vi "Prompt for Password.vi"(11 "Pipe Path":path) -> ()   [LabVIEW 2020, in "NI_SSH.lvlib" / "OpenSSH Client.lvclass"]
uses:
  <vilib>/net/SSH/Client/OpenSSH/OpenSSH Client.lvclass
  <vilib>/Subprocess/Subprocess/Subprocess.lvclass
panel:
  in  "Cancel":bool
  in  "OK":bool
  in  "Password":string="\n\n\nmz3bq.ar" caption="Password:"
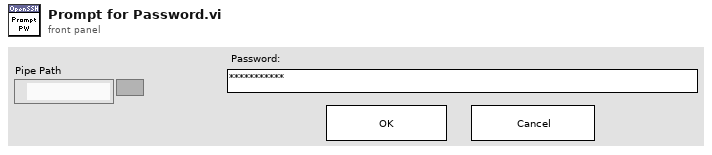
[diagram p1: front panel]
types:
  T1 = enum32{"Invalid", "Standard", "Closed", "Hidden", "Minimized", "Maximized"}
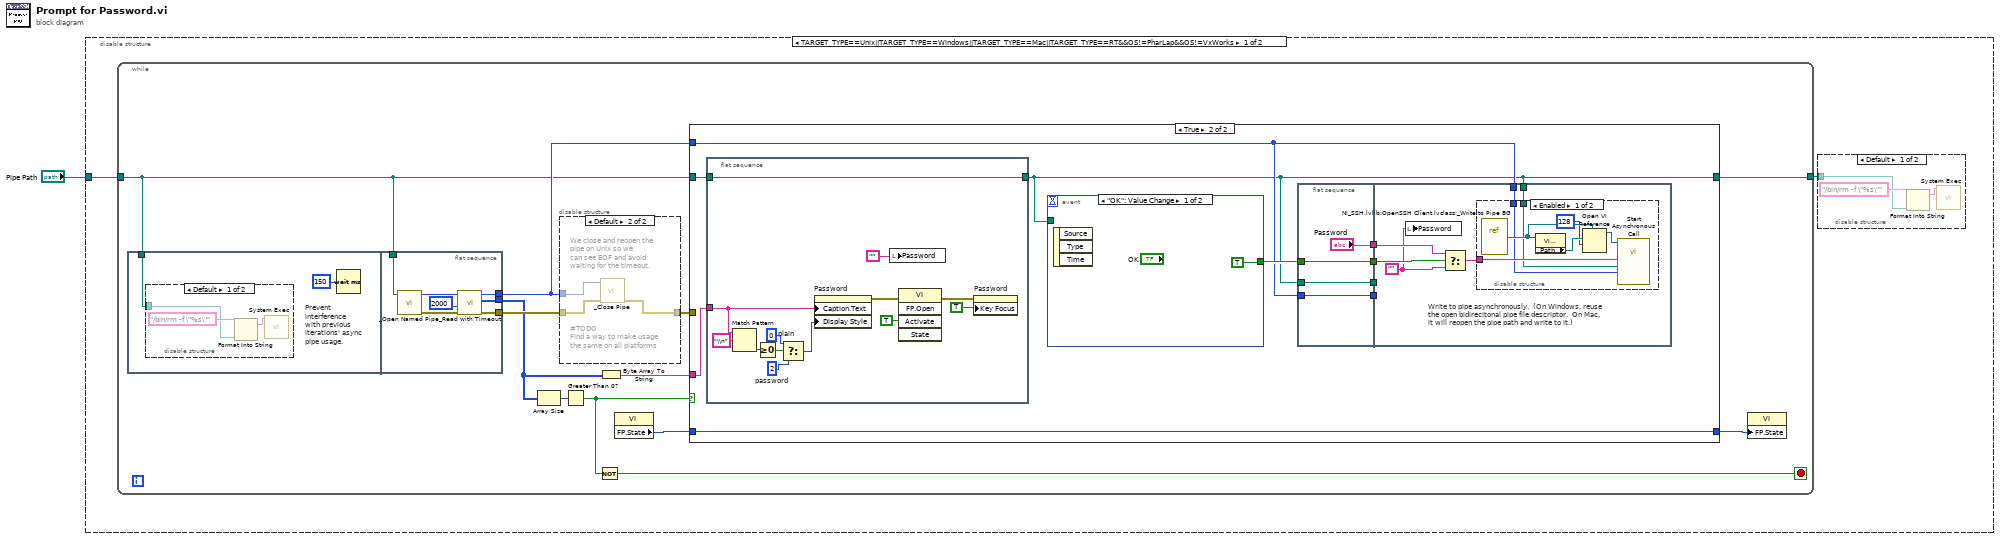
[diagram p0: block diagram]
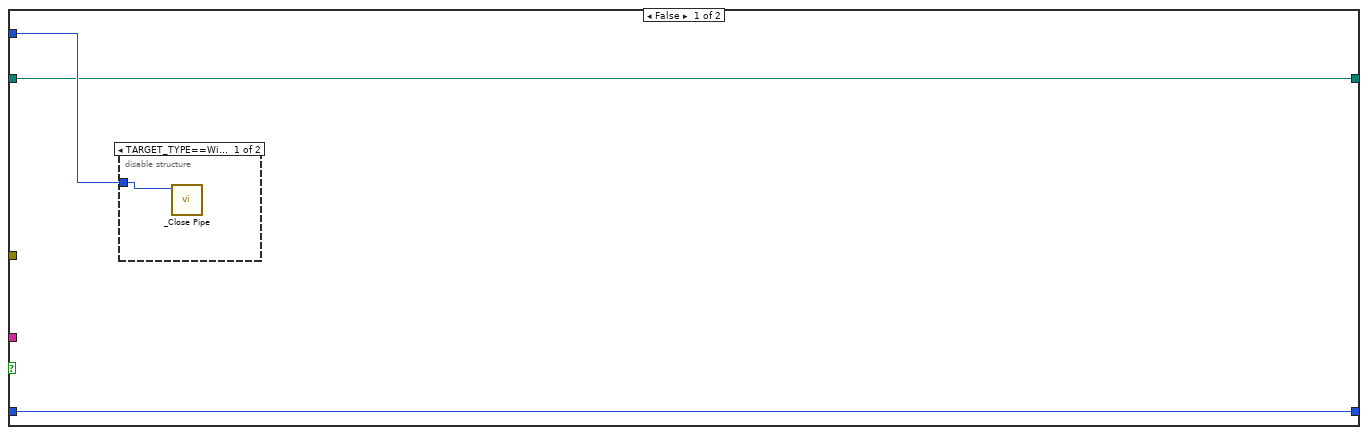
[diagram p5: hidden frame]
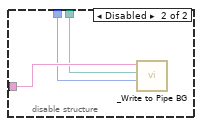
[diagram p7: hidden frame]
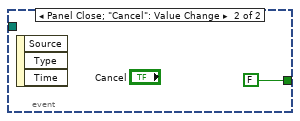
[diagram p8: hidden frame]
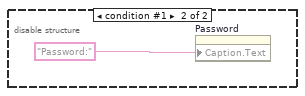
[diagram p9: hidden frame]
diagram:
  n1 = disable-structure "Conditional Disable Structure" shown="TARGET_TYPE==Unix||TARGET_TYPE==Windows||TARGET_TYPE==Mac||TARGET_TYPE==RT&&OS!=PharLap&&OS!=VxWorks" {
    disable-tunnel: "Pipe Path" -> [w3 _]
    frame condition #0 (active) {
      n2 = while {
        tunnel: w3 -> [w7]
        tunnel: [w8] -> w2
        stop <- w14 stop-if-true
        n3 = flat-sequence {
          tunnel: w7 -> [w19]
          tunnel: [w29] -> w12
          tunnel: [w28] -> w11
          tunnel: [w27] -> w10
          tunnel: w7 -> [w26]
          frame #0 {
            # "Prevent\ninterference\nwith previous\niterations' async\npipe usage."
            n4 = disable-structure shown="Default" {
              disable-tunnel: w19 -> [w21 _]
              frame condition #0 {
                n5 = Format Into String(format string="/bin/rm -f \"%s\"", w21) -> (resulting string=w22:string)  [unwired: 2 in, 1 out]
                n6 = call <vilib>:"System Exec.vi"("command line"=w22) -> ()  [unwired: 7 in, 4 out]
              }
              frame condition #1 (active) {
              }
            }
            n7 = Wait (ms)(milliseconds to wait=u32 150) -> ()  [unwired: 1 out]
          }
          frame #1 {
            n8 = call <vilib>:"_Open Named Pipe.vi"("Path"=w26) -> ("error out"=w25:errorcluster, "fd out"=w24:u64)  [unwired: 9 in]
            n9 = call <vilib>:"_Read with Timeout.vi"("error in (no error)"=w25, "timeout (ms) out"=2000, "read fd"=w24) -> ("error out 2"=w28:errorcluster, "read data"=w27:u8[], "read fd out"=w29:u64)  [unwired: 5 in, 1 out]
          }
        }
        n10 = Array Size(array=w10) -> (size(s)=w13:i32)
        n11 = disable-structure shown="Default" {
          disable-tunnel: w12 -> [_ w34]
          disable-tunnel: w11 -> [w31 w33]
          disable-tunnel: [w31 w32] -> w9
          frame condition #0 (active) {
          }
          frame condition #1 {
            # "#TODO\nFind a way to make usage\nthe same on all platforms"
            # "We close and reopen the \npipe on Unix so we\ncan see EOF and avoid\nwaiting for the timeout."
            n12 = call <vilib>:"_Close Pipe.vi"("error in"=w33, "fd"=w34) -> ("error out"=w32:errorcluster)  [unwired: 8 in, 1 out]
          }
        }
        n13 = Greater Than 0?(x=w13) -> (x > 0?=w15:bool)
        n14 = Not(x=w15) -> (.not. x?=w14:bool)
        n15 = Byte Array To String(unsigned byte array=w10) -> (string=w18:string)
        n16 = property on="Property Node" class="VI"() -> ("FP.State"=w17:T1)  [unwired: 2 in, 2 out]
        n17 = case shown="True" w15 {
          tunnel: w7 -> [w35 w48]
          tunnel: w18 -> [_ w47]
          tunnel: w17 -> [w37 w46]
          tunnel: [w37 w46] -> w16
          tunnel: w12 -> [w36 w40]
          tunnel: w9 -> [_ _]
          tunnel: [w35 w39] -> w8
          frame False {
            n18 = disable-structure shown="TARGET_TYPE==Windows||OS==Win" {
              disable-tunnel: w36 -> [w38 _]
              frame condition #0 (active) {
                n19 = call <vilib>:"_Close Pipe.vi"("fd"=w38) -> ()  [unwired: 9 in, 2 out]
              }
              frame condition #1 {
              }
            }
          }
          frame True {
            n20 = flat-sequence {
              tunnel: w48 -> [w81]
              tunnel: [w81] -> w39
              tunnel: w47 -> [w77]
              frame #0 {
                w73 = u32 0  # plain
                w72 = u32 2  # password
                n21 = Match Pattern(string=w77, regular expression="\\n") -> (offset past match=w75:i32)  [unwired: 1 in, 3 out]
                n22 = Greater Or Equal To 0?(x=w75) -> (x >= 0?=w74:bool)
                n23 = Select(t=w73, s=w74, f=w72) -> (s? t:f=w71:u32)
                n24 = property on="Password" class="Str"("Caption.Text"=w77, "Display Style"=w71) -> (error out=w79:errorcluster)  [unwired: 2 in, 1 out]
                n25 = local write "Password"("") -> ()
                n26 = invoke on="Invoke Node" class="VI" method="FP.Open"(error in=w79, "Activate"=TRUE ("Activate?")) -> (error out=w78:errorcluster)  [unwired: 3 in, 4 out]
                n27 = property on="Password" class="Str"(error in=w78, "Key Focus"=TRUE) -> ()  [unwired: 1 in, 2 out]
              }
            }
            n28 = event shown="[0] \"OK\": Value Change" {
              selector: _ -> [_ _]
              dyn-events: _ -> [_ _]
              timeout: _ -> [_ _]
              tunnel: [TRUE FALSE] -> w42
              tunnel: w39 -> [_ _]
              event "OK": Value Change {
                n29 = event-data() -> ()  [unwired: 1 in, 3 out]
              }
              event Panel Close; "Cancel": Value Change {
                n30 = event-data() -> ()  [unwired: 1 in, 3 out]
              }
            }
            n31 = flat-sequence {
              tunnel: w42 -> [w51]
              tunnel: w39 -> [w52]
              tunnel: [w52] -> w45
              tunnel: [w51] -> w44
              tunnel: ["Password"] -> w43
              tunnel: [w49] -> w41
              tunnel: w40 -> [w49]
              tunnel: w45 -> [_]
              tunnel: w44 -> [w58]
              tunnel: w43 -> [w56]
              tunnel: w41 -> [_]
              tunnel: w40 -> [w54]
              tunnel: w39 -> [w53]
              frame #0 {
              }
              frame #1 {
                w55 = ""
                # "Write to pipe asynchronously.  (On Windows, reuse\nthe open bidirecitonal pipe file descriptor.  On Mac,\nit will reopen the pipe path and write to it.)"
                n32 = local write "Password"(w55) -> ()
                n33 = Select(t=w56, s=w58, f=w55) -> (s? t:f=w57:string)
                n34 = disable-structure shown="Enabled" {
                  disable-tunnel: w57 -> [w61 w68]
                  disable-tunnel: w54 -> [w60 w66]
                  disable-tunnel: w53 -> [w59 w67]
                  frame Enabled {
                    n35 = vi-ref "NI_SSH.lvlib:OpenSSH Client.lvclass:_Write to Pipe BG.vi"() -> (w65:refnum<vi>)
                    n36 = property on="Property Node" class="VI (strict)"(reference=w65) -> ("Path"=w64:path)  [unwired: 1 in, 2 out]
                    n37 = Open VI Reference(type specifier VI Refnum (for type only)=w65, vi path=w64, options=128) -> (vi reference=w62:refnum<vi>)  [unwired: 3 in, 1 out]
                    n38 = call-by-ref "Start Asynchronous Call"(reference=w62, "fd"=w60, "path"=w59, "Password"=w61) -> ()  [unwired: 10 in, 2 out]
                  }
                  frame Disabled {
                    n39 = call <vilib>:"_Write to Pipe BG.vi"("fd"=w66, "path"=w67, "Password"=w68) -> ()  [unwired: 9 in]
                  }
                }
              }
            }
          }
        }
        n40 = property on="Property Node" class="VI"("FP.State"=w16) -> ()  [unwired: 2 in, 2 out]
      }
      n41 = disable-structure shown="Default" {
        disable-tunnel: w2 -> [w4 _]
        frame condition #0 {
          n42 = Format Into String(format string="/bin/rm -f \"%s\"", w4) -> (resulting string=w5:string)  [unwired: 2 in, 1 out]
          n43 = call <vilib>:"System Exec.vi"("command line"=w5) -> ()  [unwired: 7 in, 4 out]
        }
        frame condition #1 (active) {
        }
      }
    }
    frame condition #1 {
      n44 = property on="Password" class="Str"("Caption.Text"="Password:") -> ()  [unwired: 2 in, 2 out]
    }
  }
